vi "Write.Construct.vi"(8 "error in (no error)":errorcluster, 9 "Refs":T1[](array[typedef]) format="%.0x", 10 "Parent":T1 format="%.0x", 11 "Write in":refnum<class "Write.lvclass">) -> (0 "error out":errorcluster, 3 "Write out":refnum<class "Write.lvclass">)   [LabVIEW 2015, in "Data Access API.lvlib" / "Write.lvclass"]
uses:
  Write.lvclass
  <vilib>/NI Veristand/Custom Device API/Custom Device Item Ref.ctl
  <vilib>/NI Veristand/Custom Device API/Data Access Type.ctl
  Write.lvclass/Write.ctl
  <vilib>/NI Veristand/Custom Device API/Custom Device API.lvlib
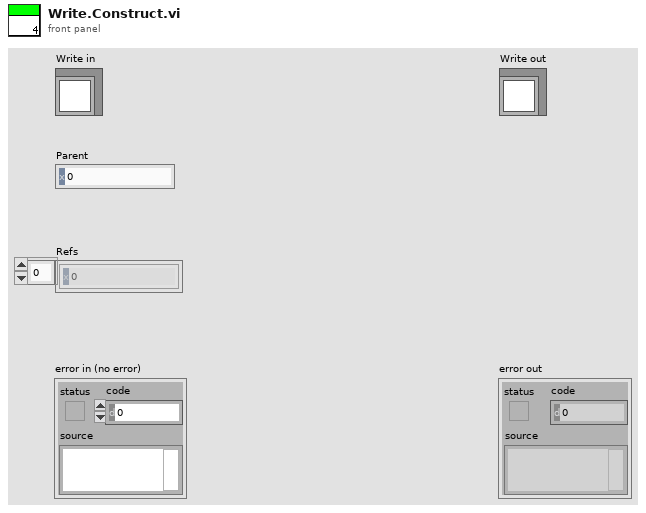
[diagram p1: front panel]
types:
  T1 = typedef "Custom Device API.lvlib/Custom Device Item Ref.ctl" = u64
  T2 = typedef "Custom Device API.lvlib/Data Access Type.ctl" = enum16{"Read", "Write"}
  T3 = typedef "Custom Device API.lvlib/Custom Device Channel.ctl" = cluster{"Type":T4, "Units":string, "Default Value":dbl, "Faultable":bool, "Scalable":bool}
  T4 = typedef "Custom Device API.lvlib/Custom Device Channel Type.ctl" = enum16{"Input", "Output"}
  T5 = typedef "Custom Device API.lvlib/Data Reference.ctl" = i32
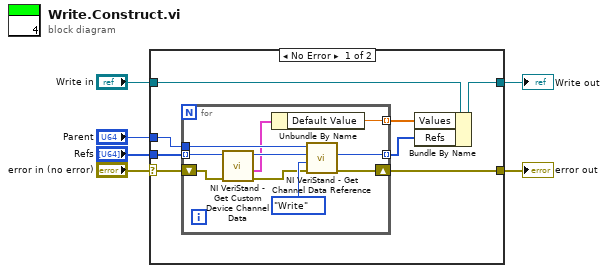
[diagram p0: block diagram]
diagram:
  n1 = case shown="No Error" "error in (no error)" {
    selector: "error in (no error)" -> [w14 w26]
    tunnel: [w13 w26] -> w5
    tunnel: [w7 w25] -> w3
    tunnel: "Write in" -> [w8 w25]
    tunnel: "Parent" -> [w12 _]
    tunnel: "Refs" -> [w11 _]
    frame No Error {
      n2 = for {
        tunnel: w12 -> [w23]
        tunnel: w11 -> [w21] mode=indexing
        shift-right: [w22] -> w13
        shift-left: w14 -> [w19]
        tunnel: [w16] -> w10 mode=indexing
        tunnel: [w15] -> w9 mode=indexing
        n3 = call <vilib>:"NI VeriStand - Get Custom Device Channel Data.vi"("error in (no error)"=w19, "Channel Ref in"=w21) -> ("error out"=w18:errorcluster, "Channel"=w17:T3, "Channel Ref out"=w20:T1)  [unwired: 4 in, 3 out]
        n4 = Unbundle By Name(w17) -> ("Default Value"=w16:dbl)
        n5 = call <vilib>:"NI VeriStand - Get Channel Data Reference.vi"("error in (no error)"=w18, "Access"=Data_Access_Type."Write", "Channel Ref in"=w20, "Device Ref in"=w23) -> ("error out"=w22:errorcluster, "Channel Data Reference"=w15:T5)  [unwired: 5 in, 1 out]
      }
      n6 = Bundle By Name(cluster=w8, "Values"=w10, "Refs"=w9) -> (w7:refnum<class "Write.lvclass">)
    }
    frame Error {
    }
  }
  "error out" <- w5
  "Write out" <- w3
